vi "MB Registers Manager Close.vi"(11 "Data Reference":T1) -> (0 "error out":errorcluster)   [LabVIEW 2019, in "NI_modbus_upd.lvlib"]
uses:
  NI_modbus_upd.lvlib
  Ctl/Data Reference.ctl
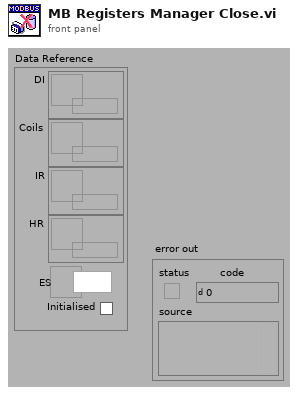
[diagram p1: front panel]
types:
  T1 = typedef "NI_modbus_upd.lvlib/Data Reference.ctl" = cluster{"DI":refnum<data-value>, "Coils":refnum<data-value>, "IR":refnum<data-value>, "HR":refnum<data-value>, "ES":refnum<data-value>, "Initialised":bool}
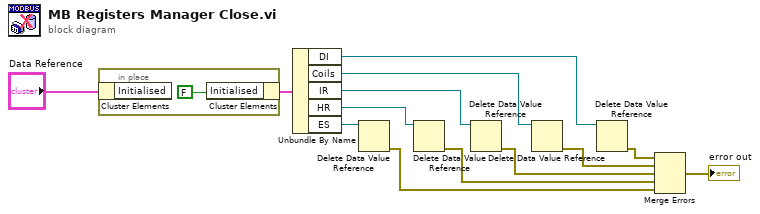
[diagram p0: block diagram]
diagram:
  n1 = in-place {
    n2 = in-place-cluster #1("Data Reference") -> ()  [unwired: 1 out]
    n3 = in-place-cluster #1("Initialised"=FALSE) -> (w3:T1)
  }
  n4 = Unbundle By Name(w3) -> ("DI"=w13:refnum<data-value>, "Coils"=w12:refnum<data-value>, "IR"=w11:refnum<data-value>, "HR"=w10:refnum<data-value>, "ES"=w2:refnum<data-value>)
  n5 = Delete Data Value Reference(data value reference=w2) -> (error out=w1:errorcluster)  [unwired: 1 in, 1 out]
  n6 = Delete Data Value Reference(data value reference=w10) -> (error out=w6:errorcluster)  [unwired: 1 in, 1 out]
  n7 = Delete Data Value Reference(data value reference=w11) -> (error out=w7:errorcluster)  [unwired: 1 in, 1 out]
  n8 = Delete Data Value Reference(data value reference=w12) -> (error out=w8:errorcluster)  [unwired: 1 in, 1 out]
  n9 = Delete Data Value Reference(data value reference=w13) -> (error out=w9:errorcluster)  [unwired: 1 in, 1 out]
  n10 = Merge Errors(w9, w8, w7, w6, w1) -> (→"error out":errorcluster)
